vi "Aero_Bal_Time_Spectra.vi"(10 "Sampling Frequency":dbl=300.0, 11 "OGI Results File":path) -> (0 "Time Trace":cluster{"Ramp Pattern":dbl[], dbl[]}[](graph), 1 "Power Spectra":cluster{dbl[], dbl[]}[](graph), 2 "Peak Amplitude":dbl[](array[numeric]), 3 "Peak Frequency":dbl[](array[numeric]))   [LabVIEW 2011]
uses:
  <vilib>/Analysis/1siggen.llb/Ramp Pattern by Samples.vi
  <vilib>/Analysis/NI_AALPro.lvlib
  <vilib>/Analysis/NI_AALBase.lvlib
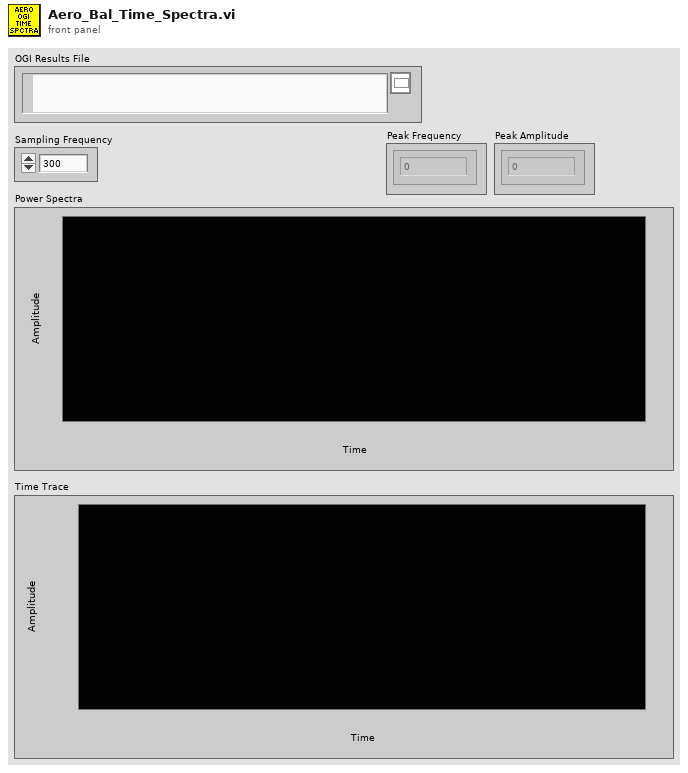
[diagram p1: front panel]
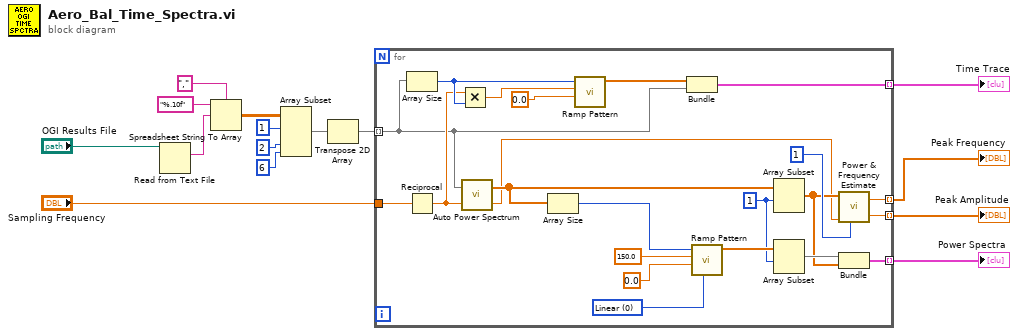
[diagram p0: block diagram]
diagram:
  n1 = Read from Text File(file (use dialog)="OGI Results File") -> (text=w15:string)  [unwired: 3 in, 3 out]
  n2 = Spreadsheet String To Array(delimiter (Tab)=",", format string="%.10f", spreadsheet string=w15) -> (array=w12:dbl[][])  [unwired: 1 in]
  n3 = Array Subset(array=w12, index (row)=1 ("index"), index (col)=2 ("index"), length (col)=6 ("length")) -> (w8:dbl[][])  [unwired: 1 in]
  n4 = Transpose 2D Array(2D array=w8) -> (transposed array=w7:dbl[][])
  n5 = for {
    tunnel: w7 -> [w19] mode=indexing
    tunnel: [w31] -> w5 mode=indexing
    tunnel: "Sampling Frequency" -> [w28]
    tunnel: [w22] -> w4 mode=indexing
    tunnel: [w20] -> w3 mode=indexing
    tunnel: [w16] -> w2 mode=indexing
    w24 = 1 ("index")
    w36 = u16 0 items=["Linear", "Logarithmic"] ("type")
    n6 = Array Size(array=w19) -> (size(s)=w33:i32)
    n7 = Reciprocal(x=w28) -> (1/x=w21:dbl)
    n8 = Multiply(x=w21, y=w33) -> (x*y=w32:dbl)
    n9 = call <vilib>:"Auto Power Spectrum.vi"("dt"=w21, "Signal (V)"=w19) -> ("df"=w17:dbl, "Power Spectrum (V^2 rms)"=w25:dbl[])
    n10 = Array Size(array=w25) -> (size(s)=w29:i32)
    n11 = call-poly <vilib>:"Ramp Pattern.vi"("start"=0.0, "end"=w32, "samples"=w33) -> ("Ramp Pattern"=w34:dbl[])  [unwired: 7 in, 1 out]
    n12 = Bundle("Ramp Pattern"=w34, w19) -> (w16:cluster{"Ramp Pattern":dbl[], dbl[]})  [unwired: 1 in]
    n13 = call-poly <vilib>:"Ramp Pattern.vi"("type"=w36, "start"=0.0, "end"=150.0, "samples"=w29) -> ("Ramp Pattern"=w26:dbl[])  [unwired: 6 in, 1 out]
    n14 = Array Subset(array=w25, index=w24) -> (w18:dbl[])  [unwired: 1 in]
    n15 = Array Subset(array=w26, index=w24) -> (w23:dbl[])  [unwired: 1 in]
    n16 = call <vilib>:"Power & Frequency Estimate.vi"("span"=1, "df"=w17, "Power Spectrum (V^2 rms)"=w18) -> ("est power peak"=w22:dbl, "est frequency peak"=w31:dbl)  [unwired: 3 in]
    n17 = Bundle(w23, w18) -> (w20:cluster{dbl[], dbl[]})  [unwired: 1 in]
  }
  "Peak Frequency" <- w5
  "Peak Amplitude" <- w4
  "Power Spectra" <- w3
  "Time Trace" <- w2
